vi "Pulse Timer.vi"(8 "error in":errorcluster, 10 "preset time (ms)":i32=1000, 11 "input":bool) -> (0 "error out":errorcluster, 2 "elapsed time (ms)":i32, 3 "output":bool)   [LabVIEW 2017, in "NI_FunctionBlock Libraries.lvlib"]
uses:
  <vilib>/functionblocks/NI_FunctionBlock Libraries.lvlib
  <vilib>/ptbypt/NI_PtbyPt.lvlib
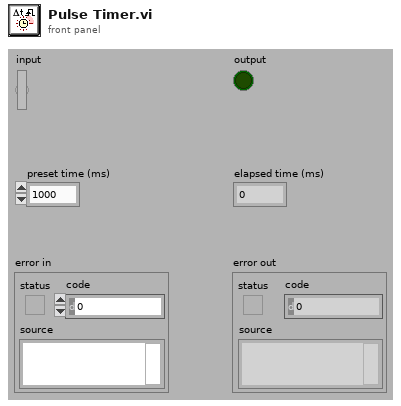
[diagram p1: front panel]
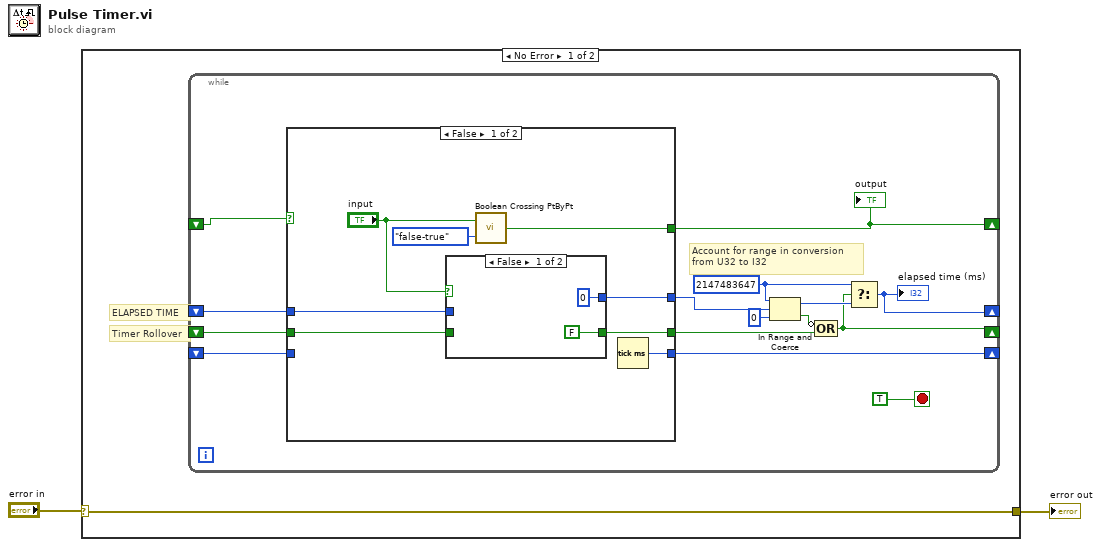
[diagram p0: block diagram]
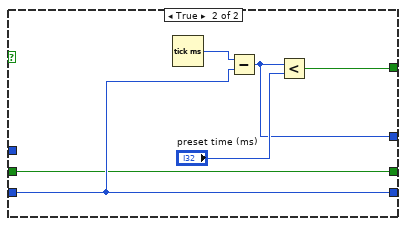
[diagram p3: hidden frame]
diagram:
  n1 = case shown="No Error" "error in" {
    selector: "error in" -> [w3 w37]
    tunnel: [w3 w37] -> w1
    frame No Error {
      # "Timer Rollover"
      # "ELAPSED TIME"
      n2 = while {
        shift-right: [w18] -> _
        shift-left: _ -> [w16]
        shift-right: [w15] -> _
        shift-left: _ -> [w14]
        shift-right: [w7] -> _
        shift-left: _ -> [w13]
        shift-right: [w6] -> _
        shift-left: _ -> [w5]
        stop <- TRUE stop-if-true
        w12 = u32 2147483647 ("upper limit")
        # "Account for range in conversion\nfrom U32 to I32"
        n3 = case shown="False" w14 {
          tunnel: [w25 w33] -> w15
          tunnel: [w23 w32] -> w8
          tunnel: [w24 w34] -> w18
          tunnel: w16 -> [_ w34]
          tunnel: w13 -> [w21 _]
          tunnel: w5 -> [w19 w31]
          tunnel: [w20 w31] -> w4
          frame False {
            n4 = case shown="False" "input" {
              tunnel: [0 ("ELAPSED TIME (ms)") w30] -> w23
              tunnel: w21 -> [_ w30]
              tunnel: [FALSE w29] -> w20
              tunnel: w19 -> [_ w29]
              frame False {
              }
              frame True {
              }
            }
            n5 = call <vilib>:"Boolean Crossing PtByPt.vi"("direction"=enum16{"either", "false-true", "true-false"}."false-true", "input"="input") -> ("crossing"=w25:bool)  [unwired: 1 in]
            n6 = Tick Count (ms)() -> (millisecond timer value=w24:u32)
          }
          frame True {
            n7 = Tick Count (ms)() -> (millisecond timer value=w36:u32)
            n8 = Subtract(x=w36, y=w34) -> (x-y=w32:u32)
            n9 = Less?(x=w32, y="preset time (ms)") -> (x < y?=w33:bool)
          }
        }
        "output" <- w15
        n10 = In Range and Coerce(upper limit=w12, x=w8, lower limit=u32 0) -> (coerced(x)=w11:u32, In Range?=w10:bool)
        n11 = Compound Arithmetic op=OR(invert w10, w4) -> (w6:bool)
        n12 = Select(t=w12, s=w6, f=w11) -> (s? t:f=w7:u32)
        "elapsed time (ms)" <- w7
      }
    }
    frame Error {
    }
  }
  "error out" <- w1
